vi "food generator.vi"(1 "Boundary Height":i8, 2 "Boundary Width":i8, 3 "Array in":refnum<vi>) -> (0 "food location":i8[](array[numeric]))   [LabVIEW 2020]
doc: "generate a food location within the border that's not on the snake"
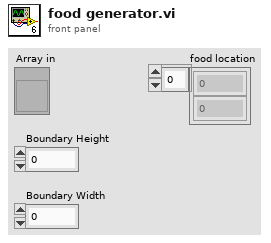
[diagram p1: front panel]
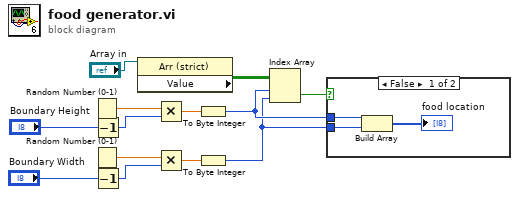
[diagram p0: block diagram]
diagram:
  n1 = Random Number (0-1)() -> (number: 0 to 1=w8:dbl)
  n2 = Random Number (0-1)() -> (number: 0 to 1=w11:dbl)
  n3 = Decrement(x="Boundary Height") -> (x-1=w2:i8)
  n4 = Decrement(x="Boundary Width") -> (x-1=w1:i8)
  n5 = property class="Arr (strict)"(reference="Array in") -> ("Value"=w12:bool[][])  [unwired: 1 in, 2 out]
  n6 = Multiply(x=w8, y=w2) -> (x*y=w9:dbl)
  n7 = Multiply(x=w11, y=w1) -> (x*y=w10:dbl)
  n8 = To Byte Integer(number=w9) -> (8bit integer=w6:i8)
  n9 = To Byte Integer(number=w10) -> (8bit integer=w5:i8)
  n10 = Index Array(array=w12, index (row)=w6, index (col)=w5) -> (element=w13:bool)
  n11 = case shown="False" w13 {
    tunnel: w6 -> [w15 _]
    tunnel: w5 -> [w14 _]
    frame False {
      n12 = Build Array(w15, w14) -> (→"food location":i8[])
    }
    frame True {
    }
  }
